vi "TCP Write (Asynchronous) - Terminated String.vi"(7 "Termination Character":string, 8 "error in":errorcluster, 9 "Timeout ms (default 50ms)":i32=50, 10 "Message to Send":string, 11 "TCP Network Connection in":refnum<k5>) -> (0 "error out":errorcluster, 3 "TCP Network Connection out":refnum<k5>)   [LabVIEW 2017, in "Communications Library.lvlib"]
doc: "Write a message to an open TCP connection."
uses:
  Communications Library.lvlib
  Error 5102 - DTACQ unit replied with an error--const.vi
  <vilib>/Utility/error.llb/Error Cluster From Error Code.vi
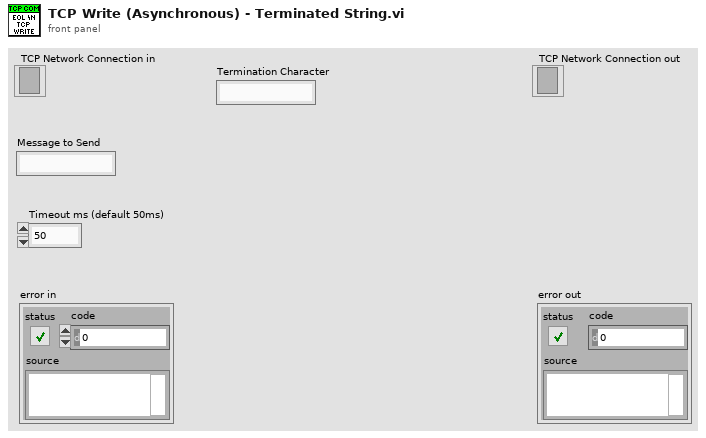
[diagram p1: front panel]
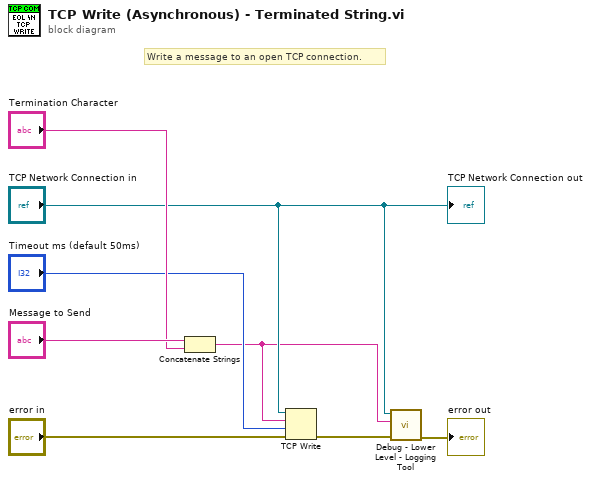
[diagram p0: block diagram]
diagram:
  # "Write a message to an open TCP connection."
  n1 = Concatenate Strings("Message to Send", "Termination Character") -> (w1:string)
  n2 = TCP Write(connection ID="TCP Network Connection in", data in=w1, error in (no error)="error in", 9:"Timeout ms (default 50ms)") -> (error out=w4:errorcluster)  [unwired: 2 out]
  n3 = call "Debug - Lower Level - Logging Tool.vi"("Error In"=w4, "Data Sent"=w1, "TCP Network Connecion In"="TCP Network Connection in") -> ("Error Out"=→"error out":errorcluster)  [unwired: 7 in, 1 out]
  "TCP Network Connection out" <- "TCP Network Connection in"
